vi "create analog task.vi"() -> (3 "task out":refnum<k21>)   [LabVIEW 2017]
doc: "SciScan 1.2 160622"
uses:
  GFG/GFGnumericGet.vi
  GFG/GFGbooleanGet.vi
  GFG/GFGstringGet.vi
  <vilib>/DAQmx/create/channels.llb/DAQmx Create Channel (AI-Voltage-Basic).vi
  GFG/GFG library.lvlib
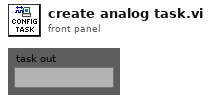
[diagram p1: front panel]
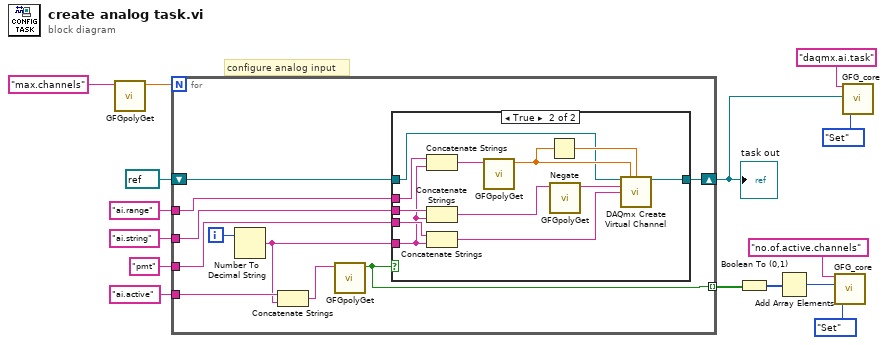
[diagram p0: block diagram]
diagram:
  # "configure analog input"
  n1 = call-poly "GFGpolyGet.vi"("Variable Name in"="max.channels") -> ("Numeric"=w9:dbl)  [unwired: 8 in, 2 out]
  n2 = for {
    N: w9 -> [_]
    shift-right: [w25] -> w1
    shift-left: refnum<k21> refnum ("task out") -> [w24]
    tunnel: "pmt" ("name to assign") -> [w19]
    tunnel: "ai.active" ("Tag in") -> [w22]
    tunnel: "ai.string" ("Tag in") -> [w18]
    tunnel: "ai.range" ("Tag in") -> [w17]
    tunnel: [w16] -> w8 mode=indexing
    i -> [w23]
    n3 = Number To Decimal String(number=w23) -> (decimal integer string=w20:string)  [unwired: 1 in]
    n4 = Concatenate Strings(w22, w20) -> (w21:string)
    n5 = call-poly "GFGpolyGet.vi"("Variable Name in"=w21) -> ("Boolean Value OUT"=w16:bool)  [unwired: 9 in, 1 out]
    n6 = case shown="True" w16 {
      tunnel: [w26 w36] -> w25
      tunnel: w24 -> [w26 w35]
      tunnel: w20 -> [_ w29]
      tunnel: w19 -> [_ w34]
      tunnel: w18 -> [_ w31]
      tunnel: w17 -> [_ w30]
      frame False {
      }
      frame True {
        n7 = Concatenate Strings(w30, w29) -> (w28:string)
        n8 = Concatenate Strings(w31, w29) -> (w32:string)
        n9 = Concatenate Strings(w34, w29) -> (w33:string)
        n10 = call-poly "GFGpolyGet.vi"("Variable Name in"=w28) -> ("Numeric"=w38:dbl)  [unwired: 8 in, 2 out]
        n11 = Negate(x=w38) -> (-x=w37:dbl)
        n12 = call-poly "GFGpolyGet.vi"("Variable Name in"=w32) -> ("String"=w27:string)  [unwired: 9 in, 1 out]
        n13 = call-poly <vilib>:"DAQmx Create Virtual Channel.vi"("task in"=w35, "maximum value"=w38, "minimum value"=w37, "physical channels"=w27, "name to assign"=w33) -> ("task out"=w36:refnum<k21>)  [unwired: 9 in, 1 out]
      }
    }
  }
  "task out" <- w1
  n14 = Boolean To (0,1)(Boolean=w8) -> (0, 1=w7:i16[])
  n15 = Add Array Elements(numeric array=w7) -> (sum=w5:i16)
  n16 = call "GFG_core.vi"("Variable Name in"="no.of.active.channels", "Variant in"=w5, "Action"=enum16{"Init", "Set", "Get"}."Set") -> ()  [unwired: 10 in, 7 out]
  n17 = call "GFG_core.vi"("Variable Name in"="daqmx.ai.task", "Variant in"=w1, "Action"=enum16{"Init", "Set", "Get"}."Set") -> ()  [unwired: 10 in, 7 out]
